vi "WaitForStabilisation.vi"(6 "Graph in":cluster{dbl[], dbl[]}, 7 "WaitTime":i32, 8 "error in":errorcluster, 9 "SampleCount":i32, 10 "Variance/Mean Trigger":dbl) -> (0 "error out":errorcluster, 2 "Values":cluster{dbl[], dbl[]})   [LabVIEW 2013]
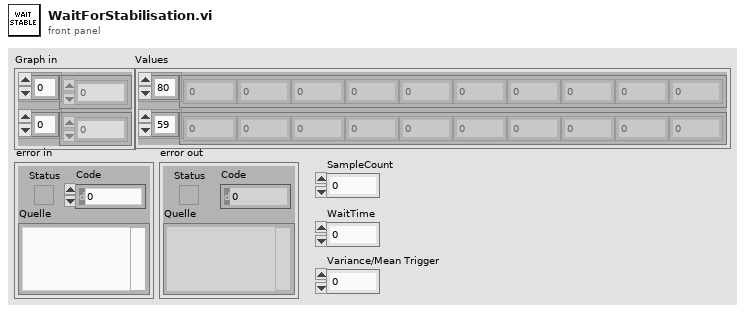
[diagram p1: front panel]
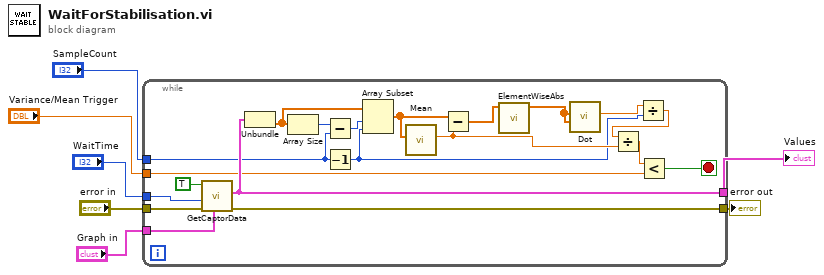
[diagram p0: block diagram]
diagram:
  n1 = while {
    tunnel: "error in" -> [w21]
    tunnel: [w20] -> w4
    tunnel: "Graph in" -> [w26]
    tunnel: [w22] -> w6
    tunnel: "SampleCount" -> [w15]
    tunnel: "Variance/Mean Trigger" -> [w17]
    tunnel: "WaitTime" -> [w19]
    stop <- w18 stop-if-true
    n2 = call "GetCaptorData.vi"("Graph in"=w26, "error in"=w21, "Length"=w19, "ON"=TRUE) -> ("error out"=w20:errorcluster, "Values"=w22:cluster{dbl[], dbl[]})  [unwired: 6 in]
    n3 = Unbundle(w22) -> (w25:dbl[])  [unwired: 1 out]
    n4 = Array Size(array=w25) -> (size(s)=w24:i32)
    n5 = Subtract(x=w24, y=w15) -> (x-y=w23:i32)
    n6 = Decrement(x=w15) -> (x-1=w10:i32)
    n7 = Array Subset(array=w25, index=w23, length=w10) -> (w16:dbl[])
    n8 = call "Mean.vi"("Array"=w16) -> ("Mean"=w14:dbl)  [unwired: 10 in]
    n9 = Subtract(x=w16, y=w14) -> (x-y=w9:dbl[])
    n10 = call "ElementWiseAbs.vi"("Array [in]"=w9) -> ("Array[out]"=w8:dbl[])  [unwired: 10 in]
    n11 = call "Dot.vi"("Points Ajustés"=w8, "Y"=w8) -> ("dot(X,Y)"=w11:dbl)  [unwired: 9 in]
    n12 = Divide(x=w11, y=w10) -> (x/y=w12:dbl)
    n13 = Divide(x=w12, y=w14) -> (x/y=w13:dbl)
    n14 = Less?(x=w13, y=w17) -> (x < y?=w18:bool)
  }
  "Values" <- w6
  "error out" <- w4
